vi "Get Value (Object).vi"(8 "error in (no error)":errorcluster, 10 "key":string, 11 "JSON Object in":refnum<class "JSON Object.lvclass">) -> (0 "error out":errorcluster, 2 "value":refnum<class "JSON Object.lvclass">)   [LabVIEW 2015, in "LVJSON.lvlib" / "JSON Object.lvclass"]
uses:
  JSON Object.lvclass
  JSON Datatype/To More Specific Type (Object).vi
  JSON Datatype/JSON Datatype.lvclass
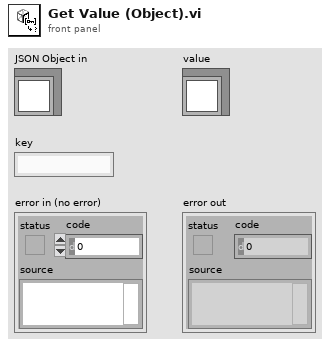
[diagram p1: front panel]
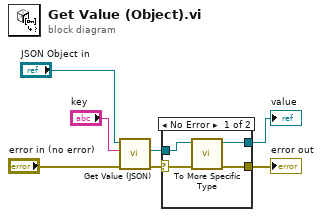
[diagram p0: block diagram]
diagram:
  n1 = call "Get Value (JSON).vi"("error in (no error)"="error in (no error)", "key"="key", "JSON Object in"="JSON Object in") -> ("error out"=w1:errorcluster, "value"=w2:refnum<class "JSON Datatype.lvclass">)  [unwired: 7 in]
  n2 = case shown="No Error" w1 {
    selector: w1 -> [w8 w12]
    tunnel: w2 -> [w10 _]
    tunnel: [w11 _] -> w3
    tunnel: [w9 w12] -> w6
    frame No Error {
      n3 = call-poly "To More Specific Type.vi"("error in (no error)"=w8, "JSON Datatype in"=w10) -> ("error out"=w9:errorcluster, "JSON Datatype out"=w11:refnum<class "JSON Object.lvclass">)  [unwired: 8 in]
    }
    frame Error {
    }
  }
  "error out" <- w6
  "value" <- w3
